vi "process incoming messages.vi"(8 "error in":errorcluster, 10 "loop comms in":T13, 11 "control loop data in":T1) -> (0 "error out":errorcluster, 3 "control loop data out":T1)   [LabVIEW 2013, in "main engine.lvlib"]
uses:
  main engine.lvlib
  control loop data.ctl
  <vilib>/NI/Tag Bus/table/data table.ctl
  engine run schedule.ctl
  engine decimation schedule.ctl
  full module data.ctl
  <vilib>/NI/DCAF Module Framework/runtime/TBM module execution interface.lvclass
  module run state.ctl
  async executor/asynchronous executor reference.ctl
  async executor/async message to executor.ctl
  Runtime/async command notification.ctl
  Runtime/async error info.ctl
  <vilib>/NI/DCAF Module Framework/runtime/error classification.ctl
  <vilib>/NI/DCAF Module Framework/module configuration/TBM module configuration.lvclass
  module method data.ctl
  <vilib>/NI/Tag Bus/table/transfer specification.ctl
  <vilib>/NI/Tag Bus/tag/Data Type.ctl
  fault handling spec.ctl
  Configuration/Error Actions.ctl
  loop comms.ctl
  message to engine.ctl
  message request type.ctl
  message from engine.ctl
  message response type.ctl
  <vilib>/NI/Tag Bus/table/data table.lvlib
  <vilib>/NI/Tag Bus/tag/tag descriptor.lvclass
  Configuration/Standard Engine Configuration.lvclass
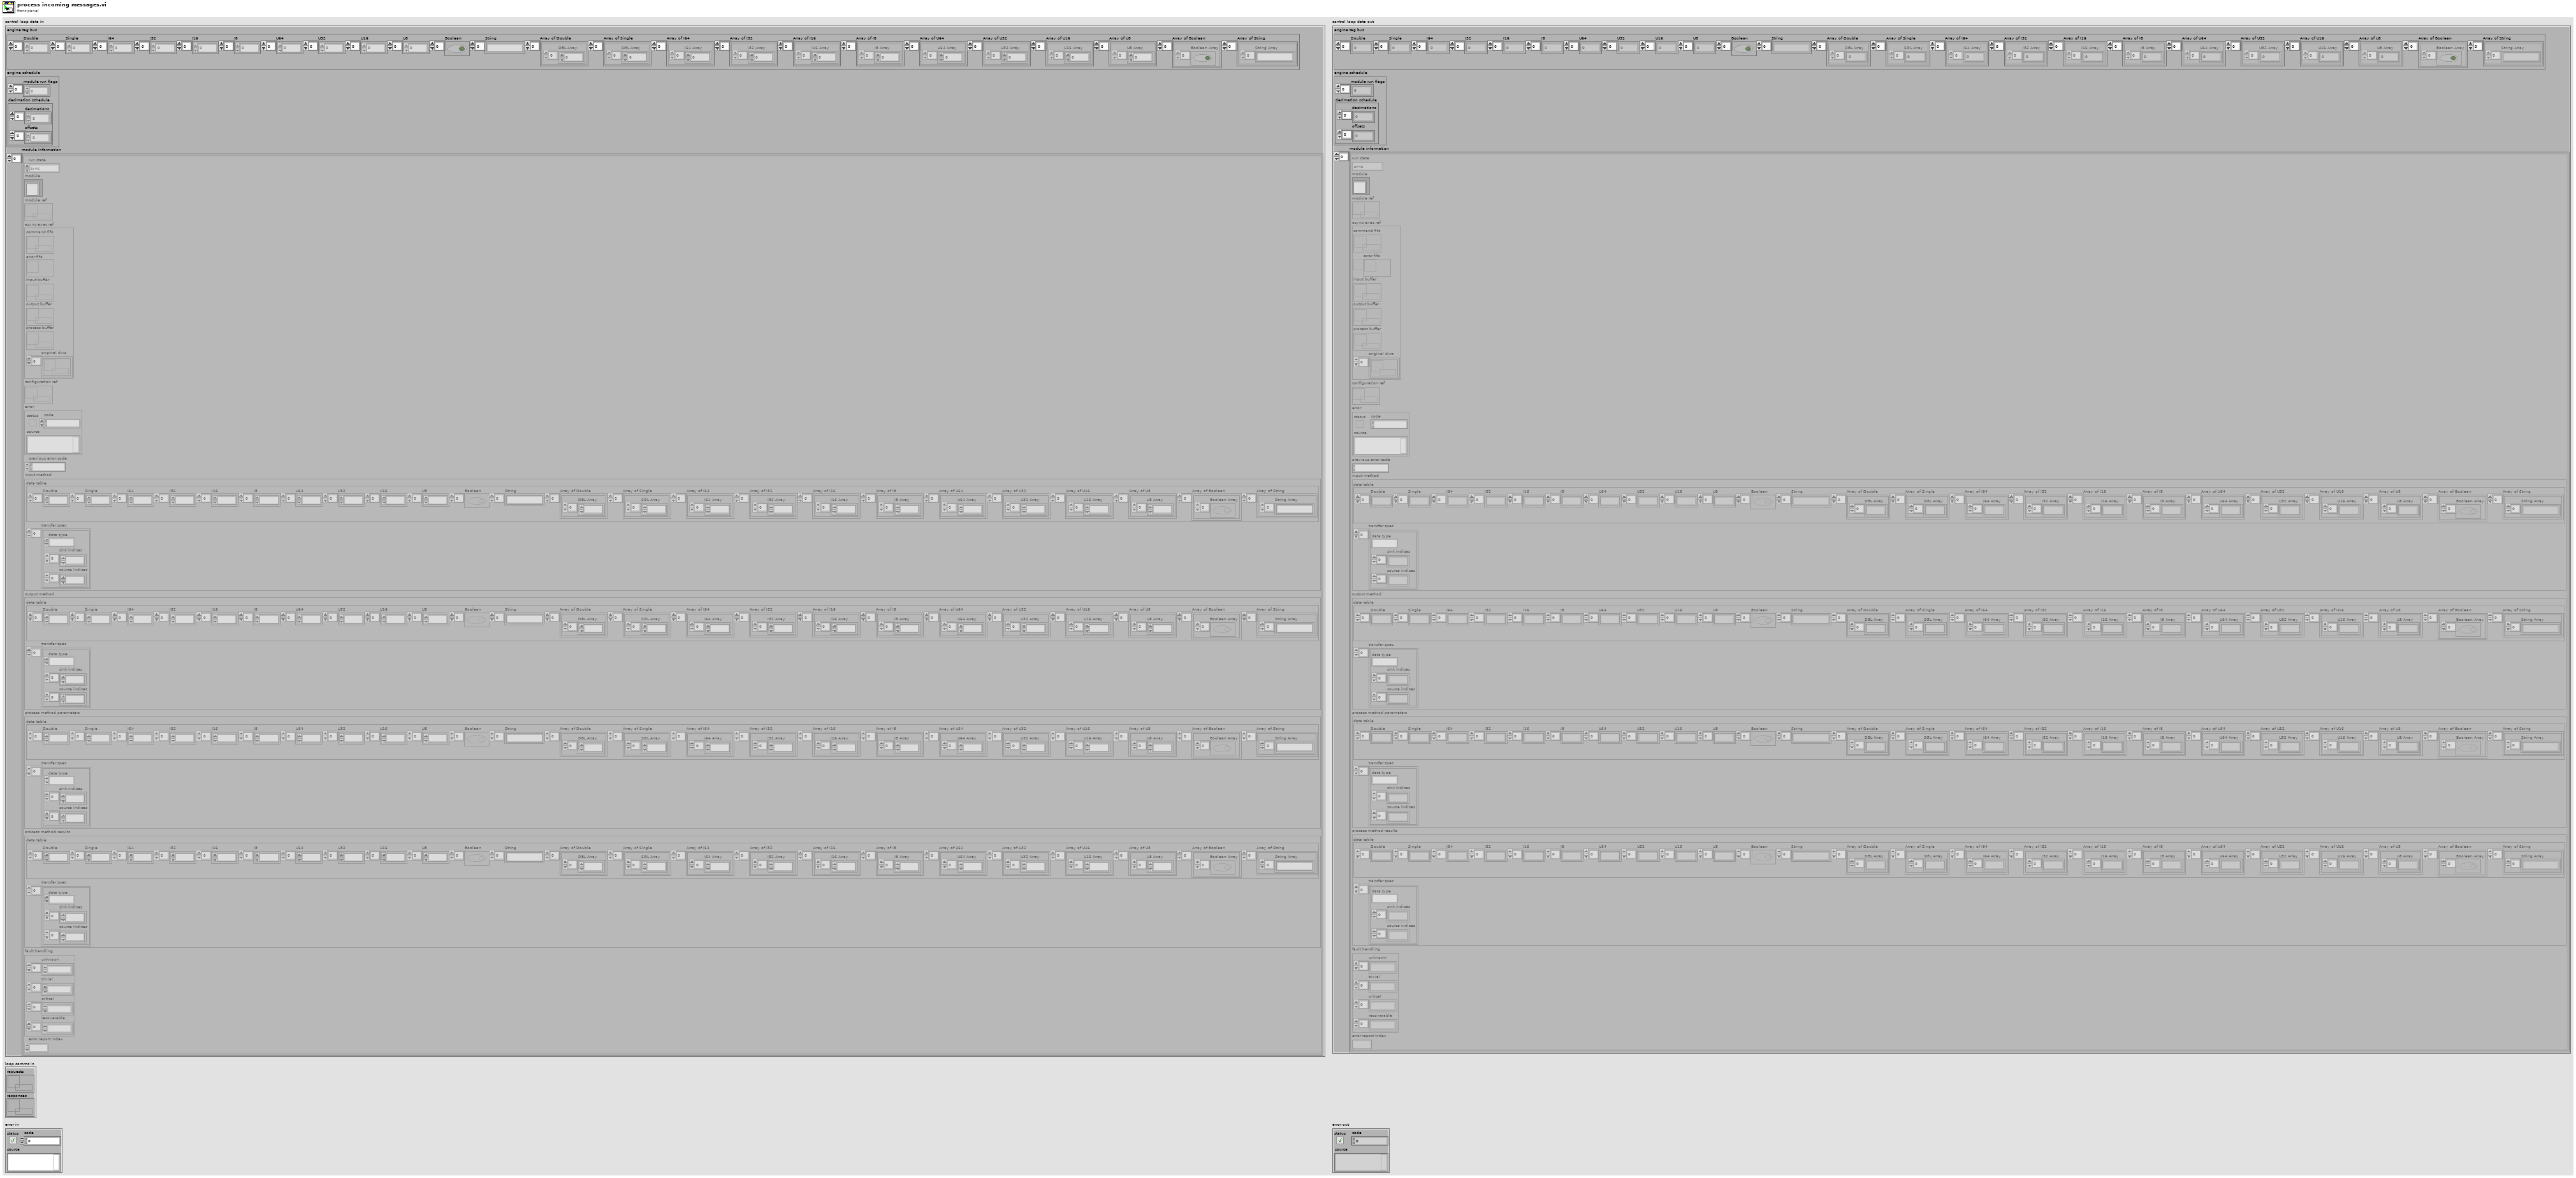
[diagram p1: front panel]
types:
  T1 = typedef "main engine.lvlib/control loop data.ctl" = cluster{"engine tag bus":T2, "engine schedule":T3, "module information":T5[]}
  T2 = typedef "tag bus.lvlib/data table.lvlib/data table.ctl" = cluster{"Double":dbl[], "Single":sgl[], "I64":i64[], "I32":i32[], "I16":i16[], "I8":i8[], "U64":u64[], "U32":u32[], "U16":u16[], "U8":u8[], "Boolean":bool[], "String":string[], "Array of Double":cluster{"DBL Array":dbl[]}[], "Array of Single":cluster{"SGL Array":sgl[]}[], "Array of I64":cluster{"I64 Array":i64[]}[], "Array of I32":cluster{"I32 Array":i32[]}[], "Array of I16":cluster{"I16 Array":i16[]}[], "Array of I8":cluster{"I8 Array":i8[]}[], "Array of U64":cluster{"U64 Array":u64[]}[], "Array of U32":cluster{"U32 Array":u32[]}[], "Array of U16":cluster{"U16 Array":u16[]}[], "Array of U8":cluster{"U8 Array":u8[]}[], "Array of Boolean":cluster{"Boolean Array":bool[]}[], "Array of String":cluster{"String Array":string[]}[]}
  T3 = typedef "main engine.lvlib/engine run schedule.ctl" = cluster{"module run flags":u8[], "decimation schedule":T4}
  T4 = typedef "main engine.lvlib/engine decimation schedule.ctl" = cluster{"decimations":u16[], "offsets":u16[]}
  T5 = typedef "main engine.lvlib/full module data.ctl" = cluster{"run state":T6, "module":refnum<class "TBM module execution interface.lvclass">, "module ref":refnum<data-value>, "async exec ref":T7, "configuration ref":refnum<data-value>, "error":errorcluster, "previous error code":i32, "input method":T8, "output method":T8, "process method parameters":T8, "process method results":T8, "fault handling":T11, "error report index ":i32}
  T6 = typedef "main engine.lvlib/module run state.ctl" = enum16{"sync", "async"}
  T7 = typedef "main engine.lvlib/asynchronous executor reference.ctl" = cluster{"command fifo":refnum<k33>, "error fifo":refnum<k33>, "input buffer":refnum<k33>, "output buffer":refnum<k33>, "process buffer":refnum<k33>, "original dvrs":refnum<data-value>[]}
  T8 = typedef "main engine.lvlib/module method data.ctl" = cluster{"data table":T2, "transfer spec":T9[]}
  T9 = typedef "tag bus.lvlib/data table.lvlib/transfer specification.ctl" = cluster{"data type":T10, "sink indices":i32[], "source indices":i32[]}
  T10 = typedef "tag bus.lvlib/tag descriptor.lvclass/Data Type.ctl" = enum16{"Double", "Single", "I64", "I32", "I16", "I8", "U64", "U32", "U16", "U8", "Boolean", "String", "Array of Double", "Array of Single", "Array of I64", "Array of I32", "Array of I16", "Array of I8", "Array of U64", "Array of U32", "Array of U16", "Array of U8", "Array of Boolean", "Array of String"}
  T11 = typedef "main engine.lvlib/fault handling spec.ctl" = cluster{"unknown":T12[], "trivial":T12[], "critical":T12[], "recoverable":T12[]}
  T12 = typedef "Standard Engine Configuration.lvclass/Error Actions.ctl" = enum16{"Clear", "Notify", "Stop Component", "Stop Engine", "Safe State", "Attempt Recovery"}
  T13 = typedef "main engine.lvlib/loop comms.ctl" = cluster{"requests":refnum<k33>, "responses":refnum<k33>}
  T14 = typedef "main engine.lvlib/message request type.ctl" = enum8{"set value", "disable module", "enable module"}
  T15 = typedef "main engine.lvlib/message response type.ctl" = enum8{"ok", "error"}
  T16 = typedef "main engine.lvlib/message from engine.ctl" = cluster{"response type":T15, "message ID":u8, "error code":i32}
  T17 = typedef "main engine.lvlib/message to engine.ctl" = cluster{"request type":T14, "message ID":u8, "message field 1":u64, "message field 2":u64, "message field 3":u64, "message field 4":u64}
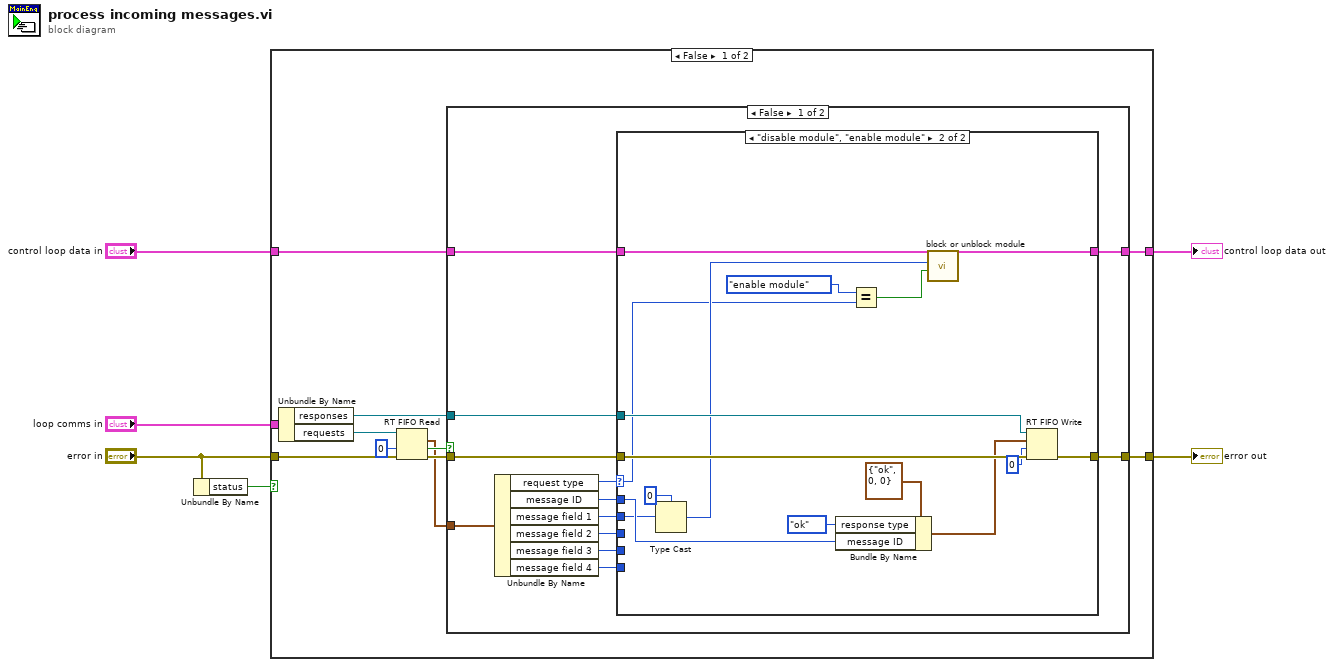
[diagram p0: block diagram]
diagram:
  n1 = Unbundle By Name("error in") -> ("status"=w4:bool)
  n2 = case shown="False" w4 {
    tunnel: "loop comms in" -> [w17 _]
    tunnel: "error in" -> [w16 w50]
    tunnel: [w11 w51] -> w3
    tunnel: "control loop data in" -> [w10 w51]
    tunnel: [w9 w50] -> w1
    frame False {
      n3 = Unbundle By Name(w17) -> ("responses"=w8:refnum<k33>, "requests"=w15:refnum<k33>)
      n4 = RT FIFO Read(0:w15, 2:0 ("timeout in ms (0)"), 3:w16) -> (9:w7:T17, 10:w12:bool, 11:w13:errorcluster)  [unwired: 1 in, 2 out]
      n5 = case shown="False" w12 {
        tunnel: w13 -> [w20 w48]
        tunnel: [w21 w49] -> w11
        tunnel: w10 -> [w22 w49]
        tunnel: [w19 w48] -> w9
        tunnel: w8 -> [w18 _]
        tunnel: w7 -> [w29 _]
        frame False {
          n6 = Unbundle By Name(w29) -> ("request type"=w28:T14, "message ID"=w27:u8, "message field 1"=w26:u64, "message field 2"=w25:u64, "message field 3"=w24:u64, "message field 4"=w23:u64)
          n7 = case shown="\"disable module\", \"enable module\"" w28 {
            selector: w28 -> [_ w34]
            tunnel: w27 -> [_ w39]
            tunnel: w26 -> [_ w37]
            tunnel: w25 -> [_ _]
            tunnel: w24 -> [_ _]
            tunnel: w23 -> [_ _]
            tunnel: w22 -> [w31 w47]
            tunnel: [w31 w46] -> w21
            tunnel: w20 -> [w30 w45]
            tunnel: [w30 w44] -> w19
            tunnel: w18 -> [_ w43]
            frame Default {
            }
            frame "disable module", "enable module" {
              n8 = Type Cast(type=0 ("timeout in ms (0)"), x=w37) -> (*(type *) &x=w35:i32)
              n9 = Bundle By Name(cluster=T16 {"response type"=enum."ok", "message ID"=0, "error code"=0} ("element"), "response type"=message_response_type."ok", "message ID"=w39) -> (w40:T16)
              n10 = Equal?(x=message_request_type."enable module", y=w34) -> (x = y?=w32:bool)
              n11 = call "block or unblock module.vi"("enable?"=w32, "module index"=w35, "control loop data in in"=w47) -> ("control loop data out"=w46:T1)  [unwired: 8 in]
              n12 = RT FIFO Write(0:w43, 1:w40, 2:0 ("timeout in ms (0)"), 3:w45) -> (11:w44:errorcluster)  [unwired: 1 in, 3 out]
            }
          }
        }
        frame True {
        }
      }
    }
    frame True {
    }
  }
  "error out" <- w1
  "control loop data out" <- w3
